vi "Q-1.vi"(0 "Application_Directory":path, 11 "Error_In":errorcluster) -> (15 "Error_Out":errorcluster)   [LabVIEW 2021]
doc: "This is a VI work as one of the front panel of the Game, asking the user First question."
uses:
  Controls/State.ctl
  Controls/Bool_Button.ctl
panel:
  in  "Home":T1=TRUE
  in  "Back?":T1=TRUE
  in  "Blue":bool
  in  "Yellow":bool
  in  "Green":bool
  in  "Red":bool
  # "Ah, dear seeker, to unlock the secrets of you,\nI must first understand the colors that resonate with your soul."
  # "Which is your favorite color?"
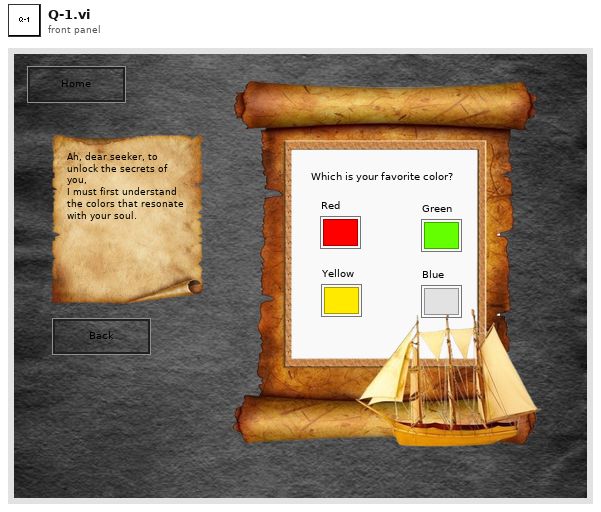
[diagram p1: front panel]
types:
  T1 = typedef "Bool_Button.ctl" = bool
  T2 = enum32{"Invalid", "Standard", "Closed", "Hidden", "Minimized", "Maximized"}
  T3 = typedef "State.ctl" = enum16{"Close", "Password_Popup", "Start_Popup", "Wizard_Msg", "Get_Name_DoB", "Lucky_Number", "Q-1", "Q-2", "Q-3", "Nature_of_the_Person"}
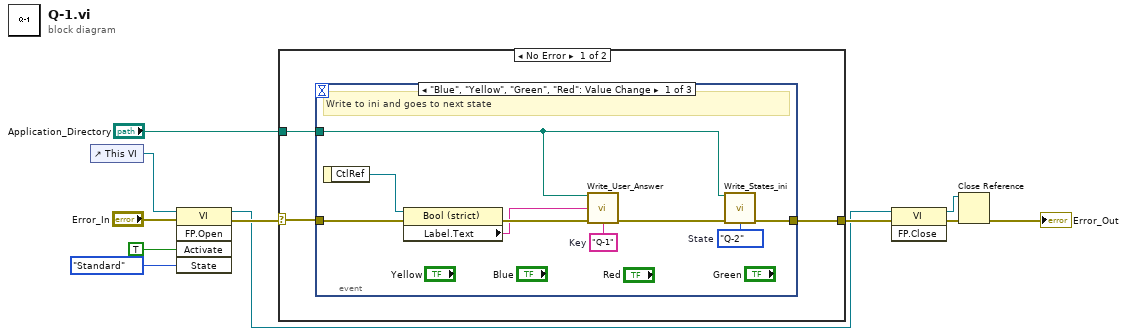
[diagram p0: block diagram]
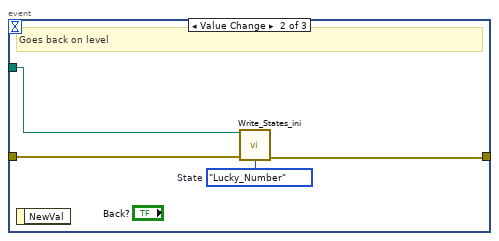
[diagram p2: hidden frame]
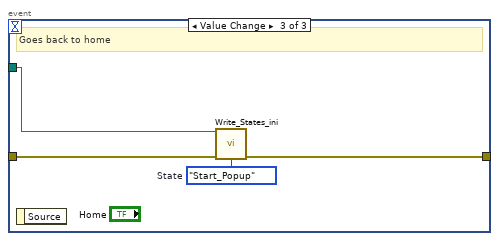
[diagram p3: hidden frame]
diagram:
  n1 = control-ref of="This VI"() -> (w9:refnum<vi>)
  n2 = invoke class="VI" method="FP.Open"(reference=w9, error in="Error_In", "Activate"=TRUE ("Activate?"), "State"=T2."Standard") -> (reference out=w1:refnum<vi>, error out=w10:errorcluster)  [unwired: 1 in, 3 out]
  n3 = case shown="No Error" w10 {
    selector: w10 -> [w14 w32]
    tunnel: [w13 w32] -> w3
    tunnel: "Application_Directory" -> [w12 _]
    frame No Error {
      n4 = event shown="[0] \"Blue\", \"Yellow\", \"Green\", \"Red\": Value Change" {
        selector: _ -> [_ _ _]
        dyn-events: _ -> [_ _ _]
        timeout: _ -> [_ _ _]
        tunnel: w14 -> [w22 w27 w31]
        tunnel: [w21 w26 w30] -> w13
        tunnel: w12 -> [w17 w24 w28]
        event "Blue", "Yellow", "Green", "Red": Value Change {
          w16 = "Q-1"  # Key
          w20 = State."Q-2"  # State
          # "Write to ini and goes to next state"
          n5 = event-data() -> ("CtlRef"=w23:refnum<vi>)  [unwired: 1 in]
          n6 = property class="Bool (strict)"(reference=w23, error in=w22) -> (error out=w19:errorcluster, "Label.Text"=w15:string)  [unwired: 1 out]
          n7 = call "Write_User_Answer.vi"("Application_Directory"=w17, "Data"=w15, "Error_In"=w19, "Key"=w16) -> ("Error_Out"=w18:errorcluster)  [unwired: 11 in]
          n8 = call "Write_States_ini.vi"("Application_Directory"=w17, "Error_In"=w18, "State"=w20) -> ("Error_Out"=w21:errorcluster)  [unwired: 12 in]
        }
        event Value Change {
          w25 = State."Lucky_Number"  # State
          # "Goes back on level"
          n9 = event-data() -> ()  [unwired: 1 in, 1 out]
          n10 = call "Write_States_ini.vi"("Application_Directory"=w24, "Error_In"=w27, "State"=w25) -> ("Error_Out"=w26:errorcluster)  [unwired: 12 in]
        }
        event Value Change {
          w29 = State."Start_Popup"  # State
          # "Goes back to home"
          n11 = event-data() -> ()  [unwired: 1 in, 1 out]
          n12 = call "Write_States_ini.vi"("Application_Directory"=w28, "Error_In"=w31, "State"=w29) -> ("Error_Out"=w30:errorcluster)  [unwired: 12 in]
        }
      }
    }
    frame Error {
    }
  }
  n13 = invoke class="VI" method="FP.Close"(reference=w1, error in=w3) -> (reference out=w4:refnum<vi>, error out=w5:errorcluster)  [unwired: 1 in, 1 out]
  n14 = Close Reference(reference=w4, error in (no error)=w5) -> (error out=→"Error_Out":errorcluster)
